vi "Update Energized.vi"(6 "Time":dbl, 8 "error in (no error)":errorcluster, 11 "2WayValve in":refnum<class "2WayValveV.lvclass">) -> (0 "error out":errorcluster, 3 "2WayValve out":refnum<class "2WayValveV.lvclass">)   [LabVIEW 2020, in "VolatusGUIElements.lvlib" / "2WayValveV.lvclass"]
uses:
  2WayValveV.lvclass
  2WayValveV.lvclass/2WayValveV.ctl
  lv-vecto/Vecto/Channel/Channel.lvclass/Channel.ctl
  lv-vecto/Vecto/Group/Value by Index.vi
  lv-vecto/Vecto/Channel/Channel.lvclass
  lv-vecto/Vecto/Vecto.lvlib
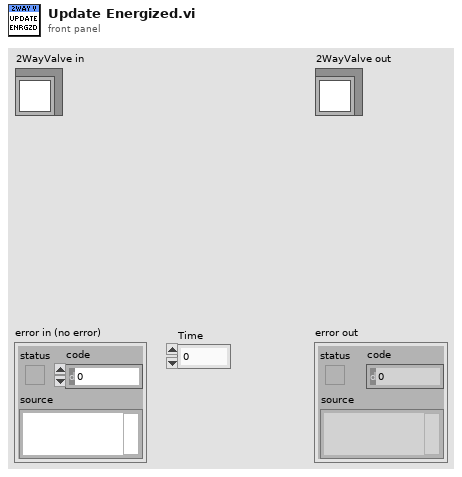
[diagram p1: front panel]
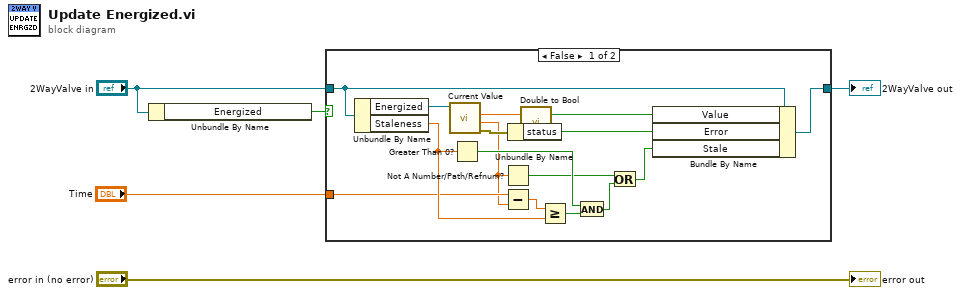
[diagram p0: block diagram]
diagram:
  n1 = Unbundle By Name("2WayValve in") -> ("Energized"=w2:bool)
  n2 = case shown="False" w2 {
    tunnel: [w10 w22] -> w4
    tunnel: "2WayValve in" -> [w11 w22]
    tunnel: "Time" -> [w12 _]
    frame False {
      n3 = Unbundle By Name(w11) -> ("Energized"=w20:refnum<class "Channel.lvclass">, "Staleness"=w15:dbl)
      n4 = call "Current Value.vi"("Channel in"=w20) -> ("error out"=w21:errorcluster, "Timestamp"=w9:dbl, "Scaled"=w19:dbl)  [unwired: 6 in, 2 out]
      n5 = Greater Than 0?(x=w15) -> (x > 0?=w13:bool)
      n6 = Not A Number/Path/Refnum?(number/path/refnum=w9) -> (NaN/Path/Refnum?=w8:bool)
      n7 = Subtract(x=w12, y=w9) -> (x-y=w18:dbl)
      n8 = Unbundle By Name(w21) -> ("status"=w16:bool)
      n9 = call "Double to Bool.vi"("Double"=w19) -> ("Bool"=w17:bool)  [unwired: 2 in]
      n10 = Greater Or Equal?(x=w18, y=w15) -> (x >= y?=w14:bool)
      n11 = And(x=w13, y=w14) -> (x .and. y?=w7:bool)
      n12 = Or(x=w8, y=w7) -> (x .or. y?=w6:bool)
      n13 = Bundle By Name(cluster=w11, "Value"=w17, "Error"=w16, "Stale"=w6) -> (w10:refnum<class "2WayValveV.lvclass">)
    }
    frame True {
      # "Energized Unused"
    }
  }
  "2WayValve out" <- w4
  "error out" <- "error in (no error)"
